vi "Init.vi"(8 "error in (no error)":errorcluster caption="错误输入（无错误）", 9 "Colleague Names":string[](array[string]), 10 "Mediator Name":string, 11 "Mediator 输入":refnum<class "Mediator.lvclass"> caption="DNL_LabVIEW Object in") -> (0 "error out":errorcluster caption="错误输出", 3 "Mediator 输出":refnum<class "Mediator.lvclass"> caption="DNL_LabVIEW Object out")   [LabVIEW 2011, in "Mediator.lvclass"]
uses:
  Mediator.lvclass
  Mediator.lvclass/Mediator.ctl
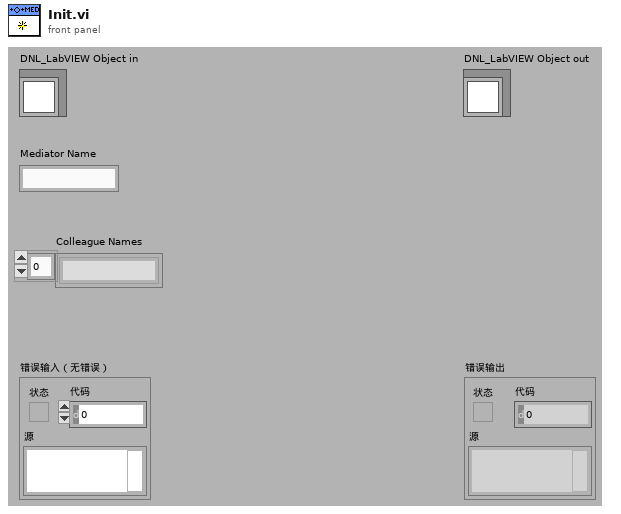
[diagram p1: front panel]
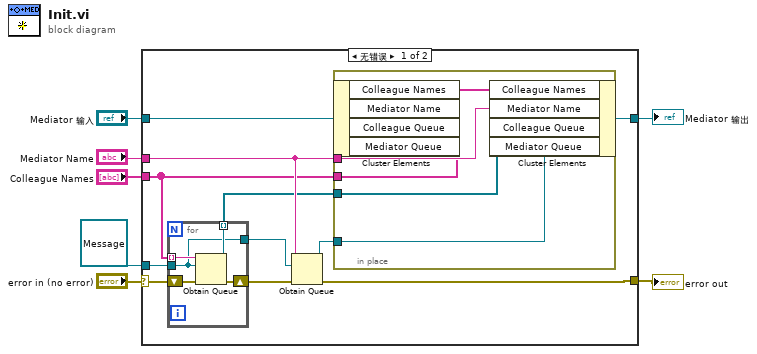
[diagram p0: block diagram]
diagram:
  n1 = case shown="无错误" "error in (no error)" {
    selector: "error in (no error)" -> [w17 w29]
    tunnel: [w11 w29] -> w6
    tunnel: [w10 w28] -> w4
    tunnel: "Mediator 输入" -> [w18 w28]
    tunnel: "Colleague Names" -> [w15 _]
    tunnel: "Mediator Name" -> [w16 _]
    tunnel: refnum<class "Message.lvclass"> refnum ("Message.lvclass") -> [w9 _]
    frame No Error {
      n2 = for {
        tunnel: w15 -> [w24] mode=indexing
        shift-right: [w26] -> w14
        shift-left: w17 -> [w27]
        tunnel: [w25] -> w12 mode=indexing
        tunnel: w9 -> [w23]
        tunnel: [w23] -> w8
        n3 = Obtain Queue(name (unnamed)=w24, element data type=w23, error in (no error)=w27) -> (queue out=w25:refnum<queue>, error out=w26:errorcluster)  [unwired: 2 in, 1 out]
      }
      n4 = Obtain Queue(name (unnamed)=w16, element data type=w8, error in (no error)=w14) -> (queue out=w13:refnum<queue>, error out=w11:errorcluster)  [unwired: 2 in, 1 out]
      n5 = in-place {
        in-place-border: w16 -> [w22]
        in-place-border: w15 -> [w21]
        in-place-border: w13 -> [w19]
        in-place-border: w12 -> [w20]
        n6 = in-place-cluster #1(w18) -> ()  [unwired: 4 out]
        n7 = in-place-cluster #1("Colleague Names"=w21, "Mediator Name"=w22, "Colleague Queue"=w20, "Mediator Queue"=w19) -> (w10:refnum<class "Mediator.lvclass">)
      }
    }
    frame Error {
    }
  }
  "error out" <- w6
  "Mediator 输出" <- w4
